vi "Start Sync.vi"(8 "error in":errorcluster, 10 "measurement plugin service in":refnum<class "Measurement Plugin Service.lvclass">, 11 "measurement service v2 in":refnum<class "Measurement Service V2.lvclass">) -> (0 "error out":errorcluster, 3 "measurement service v2 out":refnum<class "Measurement Service V2.lvclass">)   [LabVIEW 2020, in "Measurement Plugin Measurement Server.lvlib" / "Measurement Service V2.lvclass"]
uses:
  Measurement Service V2.lvclass
  C:/dev/measurementlink-labview/Source/Runtime/Measurement Plugin Measurement Server/IMeasurement Service/IMeasurement Service.lvclass
  Measurement Plugin Service/Measurement Plugin Service.lvclass
  Measurement Service V2.lvclass/Measurement Service V2.ctl
  IMeasurement Service/IMeasurement Service.lvclass
  Measurement Plugin Measurement Service Base V2/RPC Service/MeasurementService/MeasurementServiceBaseV2.lvclass
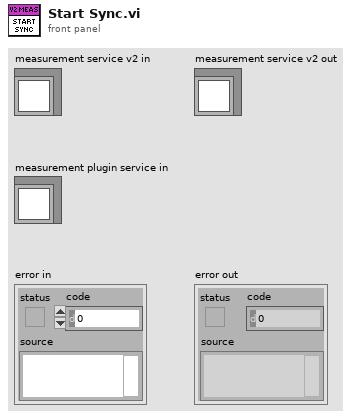
[diagram p1: front panel]
types:
  T1 = typedef "grpc-lvsupport-release.lvlib/grpcId.ctl" = u64
  T2 = typedef "Measurement Plugin Measurement Server.lvlib/Get Metadata Response.ctl" = cluster{"measurement details":T3, "measurement signature":T4, "user interface details":T9[]}
  T3 = typedef "Measurement Plugin Measurement Server.lvlib/Measurement Details.ctl" = cluster{"display name":string, "version":string}
  T4 = typedef "Measurement Plugin Measurement Server.lvlib/Measurement Signature.ctl" = cluster{"configuration parameters message type":string, "configuration parameters":T5[], "configuration defaults":T7, "outputs message type":string, "outputs":T8[]}
  T5 = typedef "Measurement Plugin Measurement Server.lvlib/Configuration Parameter.ctl" = cluster{"field number":i32, "type":i32, "name":string, "repeated":bool, "annotations":T6[], "message type":string}
  T6 = typedef "Measurement Plugin Measurement Server.lvlib/Parameter Annotations Entry.ctl" = cluster{"key":string, "value":string}
  T7 = typedef "grpc-lvsupport-release.lvlib/Any.ctl" = cluster{"Type Url":string, "Bytes":u8[]}
  T8 = typedef "Measurement Plugin Measurement Server.lvlib/Output Parameter.ctl" = cluster{"field number":i32, "type":i32, "name":string, "repeated":bool, "annotations":T6[], "message type":string}
  T9 = typedef "Measurement Plugin Measurement Server.lvlib/User Interface Details.ctl" = cluster{"file url":string}
  T10 = typedef "Measurement Plugin Measurement Service Base V2.lvlib/ni_measurementlink_measurement_v2_MeasureRequest.ctl" = cluster{"configuration_parameters":T11, "pin_map_context":T12}
  T11 = typedef "Measurement Plugin Measurement Service Base V2.lvlib/google_protobuf_Any.ctl" = cluster{"type_url":string, "value":u8[]}
  T12 = typedef "Measurement Plugin Measurement Service Base V2.lvlib/ni_measurementlink_PinMapContext.ctl" = cluster{"pin_map_id":string, "sites":i32[]}
  T13 = typedef "Measurement Plugin Measurement Server.lvlib/Measure Response.ctl" = cluster{"outputs":T14}
  T14 = typedef "Measurement Plugin Measurement Server Internal.lvlib/google_protobuf_Any.ctl" = cluster{"type_url":string, "value":u8[]}
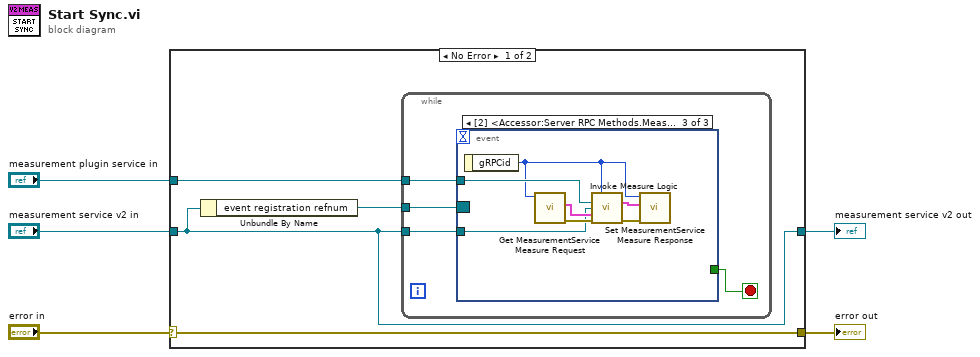
[diagram p0: block diagram]
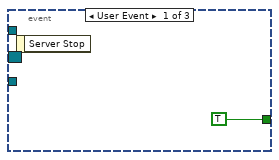
[diagram p2: hidden frame]
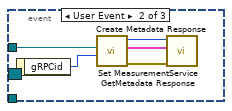
[diagram p3: hidden frame]
diagram:
  n1 = case shown="No Error" "error in" {
    selector: "error in" -> [w6 w28]
    tunnel: [w6 w28] -> w3
    tunnel: "measurement plugin service in" -> [w9 _]
    tunnel: "measurement service v2 in" -> [w8 w27]
    tunnel: [w8 w27] -> w1
    frame No Error {
      n2 = Unbundle By Name(w8) -> ("event registration refnum"=w7:refnum<event-registration>)
      n3 = while {
        tunnel: w7 -> [w13]
        tunnel: w9 -> [w12]
        tunnel: w8 -> [w10]
        stop <- w11 stop-if-true
        n4 = event "RPC Methods Event Structure" shown="[2] <Accessor:Server RPC Methods.MeasurementService Measure gRPC UE>: User Event" {
          selector: w13 -> [_ _ _]
          dyn-events: _ -> [_ _ _]
          timeout: _ -> [_ _ _]
          tunnel: [TRUE _ _] -> w11
          tunnel: w12 -> [_ w16 w25]
          tunnel: w10 -> [_ _ w20]
          event User Event {
            n5 = event-data() -> ()  [unwired: 1 in, 1 out]
          }
          event User Event {
            n6 = event-data() -> ("gRPCid"=w17:T1)  [unwired: 1 in]
            n7 = call "Create Metadata Response.vi"("gRPC ID"=w17, "measurement plugin service in"=w16) -> ("error out"=w19:errorcluster, "get metadata response"=w15:T2, "gRPC ID out"=w18:T1)  [unwired: 7 in]
            n8 = call "Set MeasurementService GetMetadata Response.vi"("error in (no error)"=w19, "Message Data"=w15, "gRPCid in"=w18) -> ()  [unwired: 8 in, 1 out]
          }
          event User Event {
            n9 = event-data() -> ("gRPCid"=w21:T1)  [unwired: 1 in]
            n10 = call "Get MeasurementService Measure Request.vi"("gRPCid"=w21) -> ("error out"=w23:errorcluster, "Message Data"=w22:T10)  [unwired: 8 in, 1 out]
            n11 = call "Invoke Measure Logic.vi"("gRPC ID in"=w21, "measurement plugin service in"=w25, "measurement service in"=w20, "measure request"=w22, "error in"=w23) -> ("measure response"=w24:T13, "error out"=w26:errorcluster)  [unwired: 9 in]
            n12 = call "Set MeasurementService Measure Response.vi"("error in (no error)"=w26, "Message Data"=w24, "gRPCid in"=w21) -> ()  [unwired: 8 in, 1 out]
          }
        }
      }
    }
    frame Error {
    }
  }
  "error out" <- w3
  "measurement service v2 out" <- w1
